vi "Configure Bus Source (SPI).vi"(0 "VISA resource name":refnum<visa-resource-name>, 1 "MOSI":T3={"MOSI Source (30: Off)"=30, "MOSI Polarity (0: High)"=0} {"MOSI Polarity (0: High)" items=["Active High", "Active Low"]; "MOSI Source (30: Off)" items=["Channel 1"=0, "Channel 2"=1, "Channel 3"=2, "Channel 4"=3, "Digital Channel 0"=14, "Digital Channel 1"=15, "Digital Channel 2"=16, "Digital Channel 3"=17, "Digital Channel 4"=18, "Digital Channel 5"=19, "Digital Channel 6"=20, "Digital Channel 7"=21, "Digital Channel 8"=22, "Digital Channel 9"=23, "Digital Channel 10"=24, "Digital Channel 11"=25, "Digital Channel 12"=26, "Digital Channel 13"=27, "Digital Channel 14"=28, "Digital Channel 15"=29, "Off"=30]}, 2 "MISO":T2={"MISO Source (30: Off)"=30, "MISO Polarity (0: High)"=0} {"MISO Polarity (0: High)" items=["Active High", "Active Low"]; "MISO Source (30: Off)" items=["Channel 1"=0, "Channel 2"=1, "Channel 3"=2, "Channel 4"=3, "Digital Channel 0"=14, "Digital Channel 1"=15, "Digital Channel 2"=16, "Digital Channel 3"=17, "Digital Channel 4"=18, "Digital Channel 5"=19, "Digital Channel 6"=20, "Digital Channel 7"=21, "Digital Channel 8"=22, "Digital Channel 9"=23, "Digital Channel 10"=24, "Digital Channel 11"=25, "Digital Channel 12"=26, "Digital Channel 13"=27, "Digital Channel 14"=28, "Digital Channel 15"=29, "Off"=30]}, 5 "BUS Number (9: Bus 1)":u16(ring)=9 items=["Bus 1"=9, "Bus 2"=10, "Bus 3"=11, "Bus 4"=12], 7 "SCLK":T1 {"SCLK Polarity (0: Rising)" items=["Rising", "Falling"]; "SCLK Source (0: Channel 1)" items=["Channel 1"=0, "Channel 2"=1, "Channel 3"=2, "Channel 4"=3, "Digital Channel 0"=14, "Digital Channel 1"=15, "Digital Channel 2"=16, "Digital Channel 3"=17, "Digital Channel 4"=18, "Digital Channel 5"=19, "Digital Channel 6"=20, "Digital Channel 7"=21, "Digital Channel 8"=22, "Digital Channel 9"=23, "Digital Channel 10"=24, "Digital Channel 11"=25, "Digital Channel 12"=26, "Digital Channel 13"=27, "Digital Channel 14"=28, "Digital Channel 15"=29]}, 9 "SS":T4={"SS Source (1: Channel 2)"=1, "SS Polarity (1: Low)"=1} {"SS Polarity (1: Low)" items=["Active High", "Active Low"]; "SS Source (1: Channel 2)" items=["Channel 1"=0, "Channel 2"=1, "Channel 3"=2, "Channel 4"=3, "Digital Channel 0"=14, "Digital Channel 1"=15, "Digital Channel 2"=16, "Digital Channel 3"=17, "Digital Channel 4"=18, "Digital Channel 5"=19, "Digital Channel 6"=20, "Digital Channel 7"=21, "Digital Channel 8"=22, "Digital Channel 9"=23, "Digital Channel 10"=24, "Digital Channel 11"=25, "Digital Channel 12"=26, "Digital Channel 13"=27, "Digital Channel 14"=28, "Digital Channel 15"=29]}, 11 "error in (no error)":errorcluster, 12 "Word Size (8 Bits)":u8=8, 13 "Bit Order (0: Most Significant First)":u16(ring) items=["Most Significant First", "Least Significant First"]) -> (4 "VISA resource name out":refnum<visa-resource-name>, 15 "error out":errorcluster)   [LabVIEW 2009, in "Tektronix DPO MSO 2000 4000 Series.lvlib"]
doc: "Configures SPI bus with SS (standard 3-wire) framing settings for an oscilloscope.\n\n<B>Note:</B>\n\nFor Idle Time framing (non-standard 2-wire SPI), use <B>Configure Bus Source (SPI - Idle Time)</B> VI instead."
uses:
  <instrlib>/Tektronix DPO MSO 2000 4000 Series/Tektronix DPO MSO 2000 4000 Series.lvlib
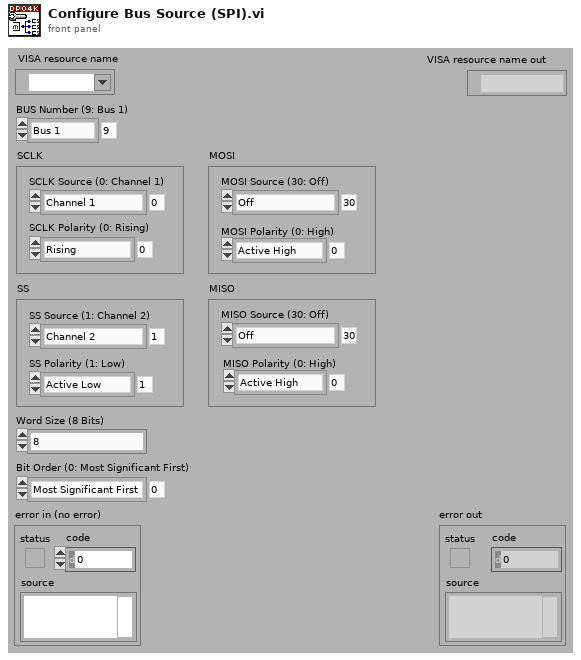
[diagram p1: front panel]
types:
  T1 = cluster{"SCLK Source (0: Channel 1)":u16, "SCLK Polarity (0: Rising)":u16}
  T2 = cluster{"MISO Source (30: Off)":u16, "MISO Polarity (0: High)":u16}
  T3 = cluster{"MOSI Source (30: Off)":u16, "MOSI Polarity (0: High)":u16}
  T4 = cluster{"SS Source (1: Channel 2)":u16, "SS Polarity (1: Low)":u16}
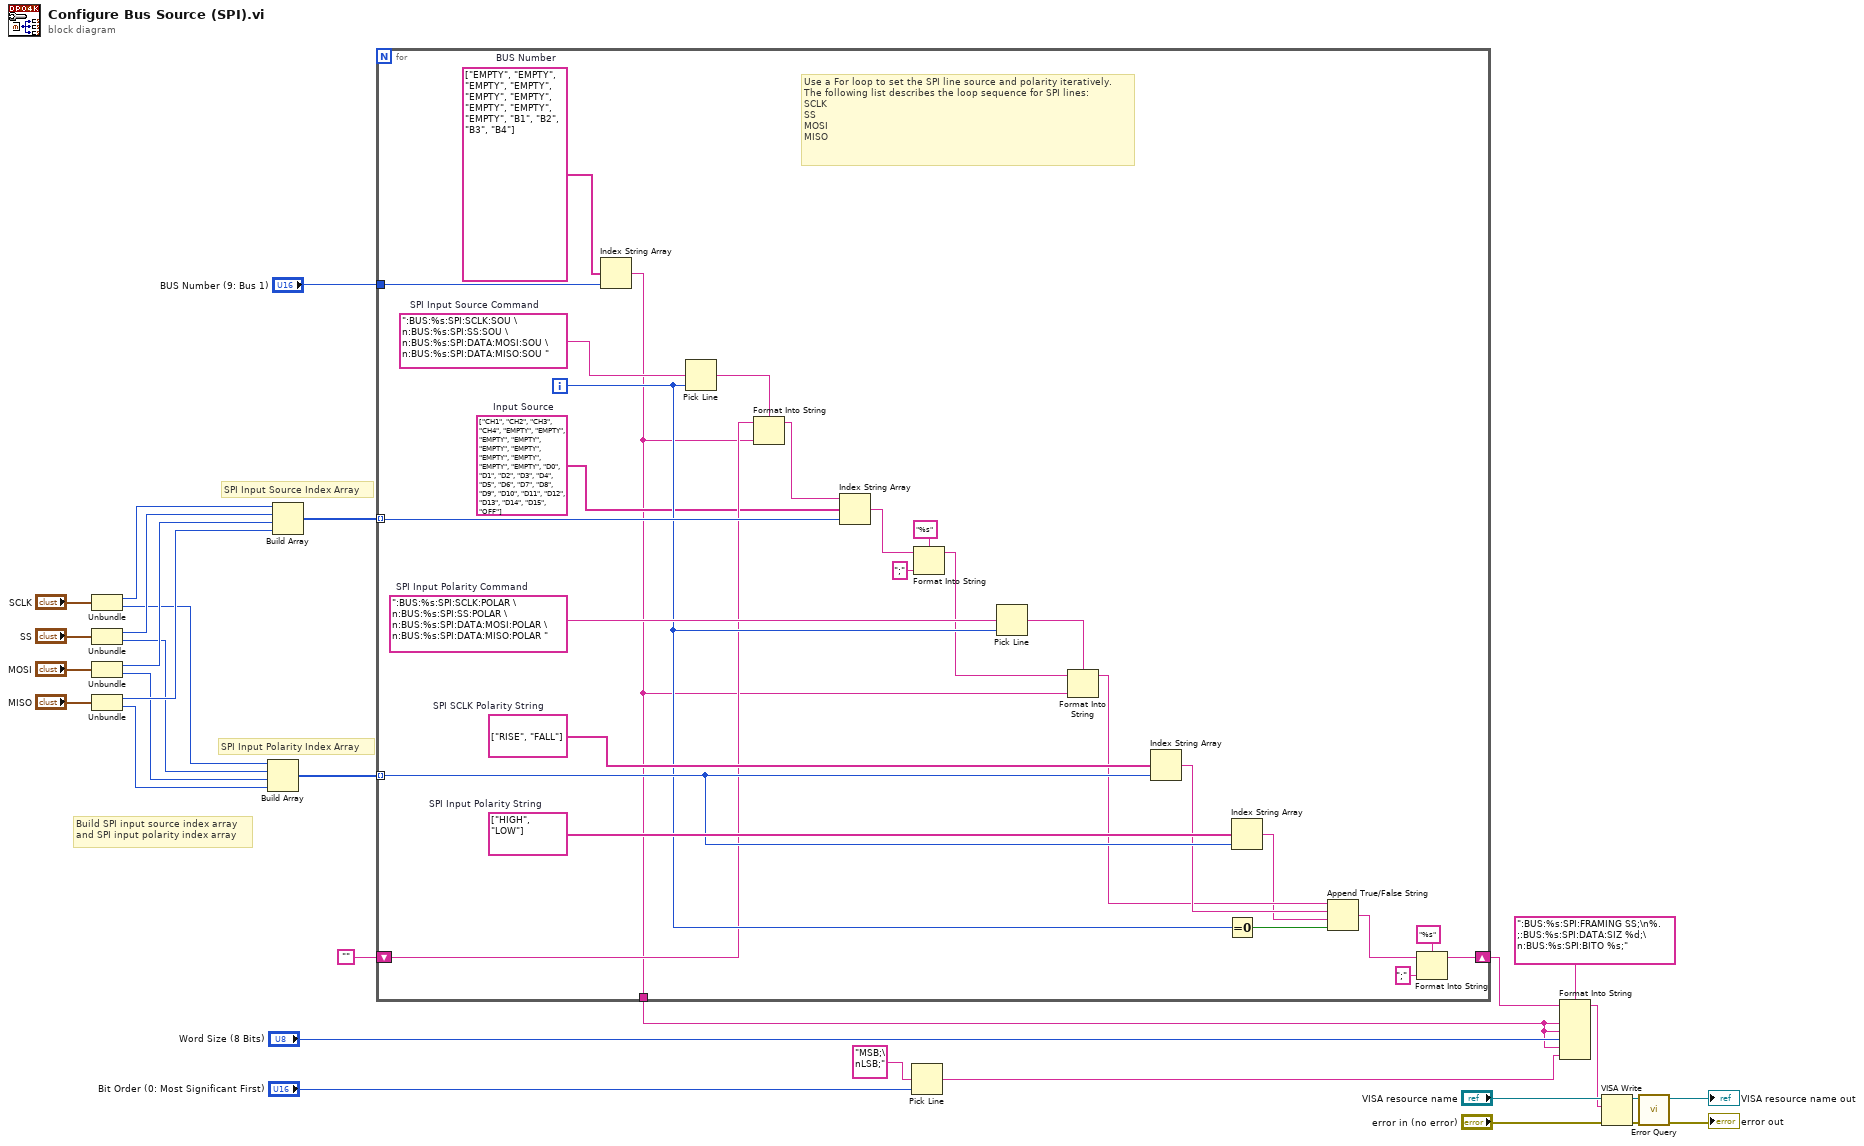
[diagram p0: block diagram]
diagram:
  # "Build SPI input source index array\nand SPI input polarity index array"
  # "SPI Input Polarity Index Array"
  # "SPI Input Source Index Array"
  n1 = Unbundle("SCLK") -> ("SCLK Source (0: Channel 1)"=w20:u16, "SCLK Polarity (0: Rising)"=w19:u16)
  n2 = Unbundle("SS") -> ("SS Source (1: Channel 2)"=w27:u16, "SS Polarity (1: Low)"=w23:u16)
  n3 = Unbundle("MOSI") -> ("MOSI Source (30: Off)"=w26:u16, "MOSI Polarity (0: High)"=w22:u16)
  n4 = Unbundle("MISO") -> ("MISO Source (30: Off)"=w25:u16, "MISO Polarity (0: High)"=w24:u16)
  n5 = Build Array(w19, w23, w22, w24) -> (w17:u16[])
  n6 = Build Array(w20, w27, w26, w25) -> (w18:u16[])
  n7 = for {
    tunnel: w18 -> [w54] mode=indexing
    tunnel: w17 -> [w48] mode=indexing
    shift-right: [w38] -> w7
    shift-left: "" -> [w35]
    tunnel: "BUS Number (9: Bus 1)" -> [w32]
    tunnel: [w31] -> w3
    i -> [w45]
    w34 = string[] ["CH1", "CH2", "CH3", "CH4", "EMPTY", "EMPTY", "EMPTY", "EMPTY", "EMPTY", "EMPTY", "EMPTY", "EMPTY", "EMPTY", "EMPTY", "D0", "D1", "D2", "D3", "D4", "D5", "D6", "D7", "D8", "D9", "D10", "D11", "D12", "D13", "D14", "D15", "OFF"]  # Input Source
    w55 = string[] ["EMPTY", "EMPTY", "EMPTY", "EMPTY", "EMPTY", "EMPTY", "EMPTY", "EMPTY", "EMPTY", "B1", "B2", "B3", "B4"]  # BUS Number
    w53 = string[] ["RISE", "FALL"]  # SPI SCLK Polarity String
    w49 = string[] ["HIGH", "LOW"]  # SPI Input Polarity String
    w56 = ":BUS:%s:SPI:SCLK:POLAR \n:BUS:%s:SPI:SS:POLAR \n:BUS:%s:SPI:DATA:MOSI:POLAR \n:BUS:%s:SPI:DATA:MISO:POLAR "  # SPI Input Polarity Command
    w57 = ":BUS:%s:SPI:SCLK:SOU \n:BUS:%s:SPI:SS:SOU \n:BUS:%s:SPI:DATA:MOSI:SOU \n:BUS:%s:SPI:DATA:MISO:SOU "  # SPI Input Source Command
    # "Use a For loop to set the SPI line source and polarity iteratively.\nThe following list describes the loop sequence for SPI lines:\nSCLK\nSS\nMOSI\nMISO"
    n8 = Index String Array(1:w32, 2:w55) -> (0:w31:string)  [unwired: 1 in]
    n9 = Pick Line(multi-line string=w57, line index=w45) -> (output string=w39:string)  [unwired: 1 in]
    n10 = Format Into String(format string=w39, initial string=w35, w31) -> (resulting string=w47:string)  [unwired: 1 in, 1 out]
    n11 = Index String Array(1:w54, 2:w34, 3:w47) -> (0:w52:string)
    n12 = Format Into String(format string="%s", initial string=w52, ";" ("input 1")) -> (resulting string=w33:string)  [unwired: 1 in, 1 out]
    n13 = Pick Line(multi-line string=w56, line index=w45) -> (output string=w46:string)  [unwired: 1 in]
    n14 = Format Into String(format string=w46, initial string=w33, w31) -> (resulting string=w42:string)  [unwired: 1 in, 1 out]
    n15 = Index String Array(1:w48, 2:w53) -> (0:w43:string)  [unwired: 1 in]
    n16 = Equal To 0?(x=w45) -> (x = 0?=w44:bool)
    n17 = Index String Array(1:w48, 2:w49) -> (0:w37:string)  [unwired: 1 in]
    n18 = Append True/False String(1:w44, 2:w37, 3:w43, 4:w42) -> (0:w36:string)
    n19 = Format Into String(format string="%s", initial string=w36, ";" ("input 1")) -> (resulting string=w38:string)  [unwired: 1 in, 1 out]
  }
  n20 = Pick Line(multi-line string="MSB;\nLSB;", line index="Bit Order (0: Most Significant First)") -> (output string=w4:string)  [unwired: 1 in]
  n21 = Format Into String(format string=":BUS:%s:SPI:FRAMING SS;\n%.;:BUS:%s:SPI:DATA:SIZ %d;\n:BUS:%s:SPI:BITO %s;" ("input 1"), initial string=w7, w3, w3, "Word Size (8 Bits)", w3, w4) -> (resulting string=w6:string)  [unwired: 1 in, 1 out]
  n22 = VISA Write(VISA resource name="VISA resource name", write buffer=w6, error in (no error)="error in (no error)") -> (VISA resource name out=w15:refnum<visa-resource-name>, error out=w14:errorcluster)  [unwired: 1 out]
  n23 = call <instrlib>:"Error Query.vi"("error in (no error)"=w14, "VISA resource name"=w15) -> ("error out"=→"error out":errorcluster, "VISA resource name out"=→"VISA resource name out":refnum<visa-resource-name>)  [unwired: 6 in, 2 out]
